vi "PM103 Peak Search Sample.vi"() -> ()   [LabVIEW 2019]
panel:
  out "Current [A]":string caption="Buffer"
  in  "Autoset":bool
  out "Active":bool
  in  "stop":bool
  # "Thorlabs Power Meter Series\n    PM103 peak search example"
  # "This example will connect the first found power meter."
  # "Connected"
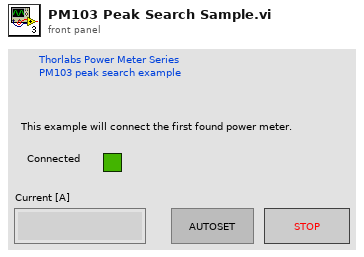
[diagram p1: front panel]
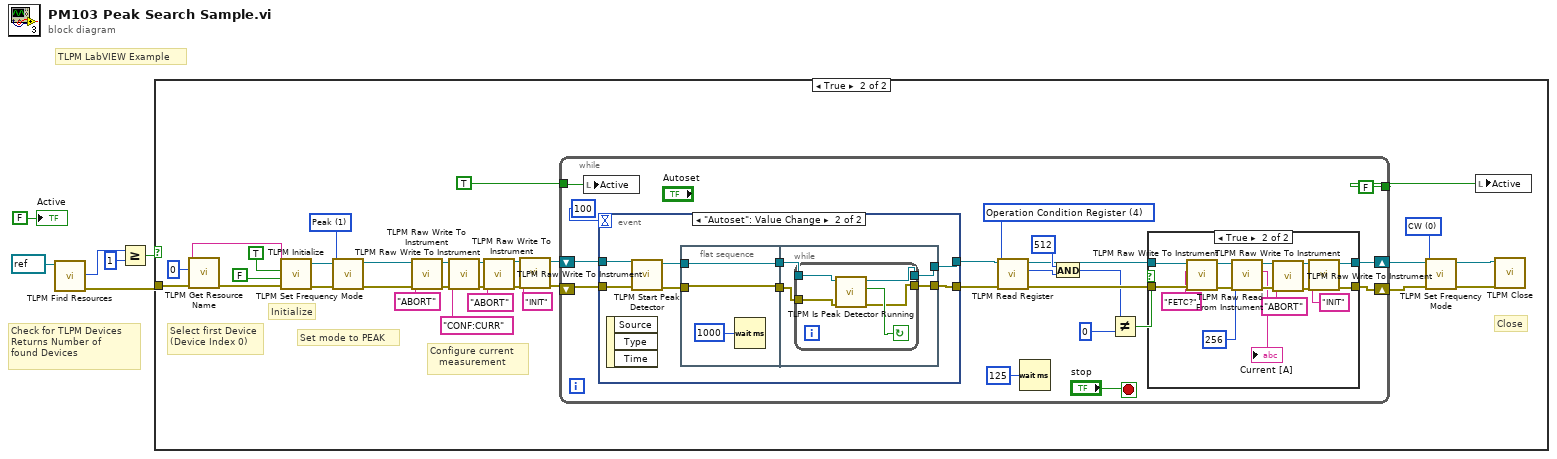
[diagram p0: block diagram]
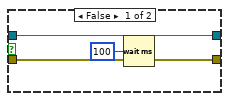
[diagram p3: hidden frame]
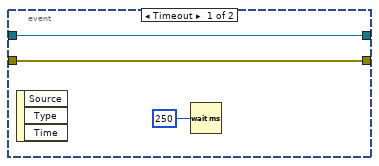
[diagram p4: hidden frame]
diagram:
  # "TLPM LabVIEW Example"
  # "Check for TLPM Devices\nReturns Number of\nfound Devices"
  n1 = call <instrlib>:"TLPM Find Resources.vi"("instrument handle"=refnum<visa-resource-name> refnum) -> ("error out"=w5:errorcluster, "Resource Count"=w3:u32)  [unwired: 8 in, 1 out]
  n2 = Greater Or Equal?(x=w3, y=u32 1) -> (x >= y?=w4:bool)
  n3 = case shown="True" w4 {
    tunnel: w5 -> [_ w34]
    frame False {
    }
    frame True {
      w7 = u16 1 items=["CW", "Peak"] ("Frequency Mode (Peak)")
      w24 = u16 0 items=["CW", "Peak"] ("Frequency Mode (Peak)")
      # "Configure current \n   measurement"
      # "Set mode to PEAK"
      # "Close"
      # "Initialize"
      # "Select first Device\n(Device Index 0)"
      n4 = call <instrlib>:"TLPM Get Resource Name.vi"("error in (no error)"=w34, "Index (0)"=u32 0 ("Device Index")) -> ("error out"=w36:errorcluster, "Resource Name"=w35:string)  [unwired: 7 in, 1 out]
      n5 = call <instrlib>:"TLPM Initialize.vi"("error in (no error)"=w36, "Reset Device (Reset Device)"=FALSE ("ID Query (Do Query)"), "ID Query (Do Query)"=TRUE, "resource name"=w35) -> ("error out"=w22:errorcluster, "instrument handle out"=w23:refnum<visa-resource-name>)  [unwired: 6 in]
      n6 = call <instrlib>:"TLPM Set Frequency Mode.vi"("error in (no error)"=w22, "Frequency Mode (Peak)"=w7, "instrument handle"=w23) -> ("error out"=w20:errorcluster, "instrument handle out"=w21:refnum<visa-resource-name>)  [unwired: 7 in]
      n7 = call <instrlib>:"TLPM Raw Write To Instrument.vi"("error in (no error)"=w20, "Command (\"*RST\")"="ABORT" ("Command (\"*RST\")"), "instrument handle"=w21) -> ("error out"=w19:errorcluster, "instrument handle out"=w13:refnum<visa-resource-name>)  [unwired: 7 in]
      n8 = call <instrlib>:"TLPM Raw Write To Instrument.vi"("error in (no error)"=w19, "Command (\"*RST\")"="CONF:CURR" ("Command (\"*RST\")"), "instrument handle"=w13) -> ("error out"=w18:errorcluster, "instrument handle out"=w12:refnum<visa-resource-name>)  [unwired: 7 in]
      n9 = call <instrlib>:"TLPM Raw Write To Instrument.vi"("error in (no error)"=w18, "Command (\"*RST\")"="ABORT" ("Command (\"*RST\")"), "instrument handle"=w12) -> ("error out"=w17:errorcluster, "instrument handle out"=w14:refnum<visa-resource-name>)  [unwired: 7 in]
      n10 = call <instrlib>:"TLPM Raw Write To Instrument.vi"("error in (no error)"=w17, "Command (\"*RST\")"="INIT" ("Command (\"*RST\")"), "instrument handle"=w14) -> ("error out"=w16:errorcluster, "instrument handle out"=w15:refnum<visa-resource-name>)  [unwired: 7 in]
      n11 = while {
        shift-right: [w42] -> w28
        shift-left: w15 -> [w50]
        shift-right: [w41] -> w27
        shift-left: w16 -> [w49]
        tunnel: [FALSE ("Active")] -> w32
        tunnel: TRUE ("Active") -> [w52]
        stop <- "stop" stop-if-true
        w48 = i16 4 items=["Status Byte Register"=0, "Service Request Enable"=1, "Standard Event Status Register"=2, "Standard Event Enable"=3, "Measurement Condition Register"=14, "Measurement Event Register"=15, "Measurement Event Enable Register"=16, "Measurement Positive Transition Filter"=17, "Measurement Negative Transition Filter"=18, "Operation Condition Register"=4, "Operation Event Register"=5, "Operation Event Enable Register"=6, "Operation Positive Transition Filter"=7, "Operation Negative Transition Filter"=8, "Questionable Condition Register"=9, "Questionable Event Register"=10, "Questionable Event Enable Register"=11, "Questionable Positive Transition Filter"=12, "Questionable Negative Transition Filter"=13, "Auxiliary Condition Register"=19, "Auxiliary Event Register"=20, "Auxiliary Event Enable Register"=21, "Auxiliary Positive Transition Filter"=22, "Auxiliary Negative Transition Filter"=23] ("Register ID (Status Byte Register)")
        n12 = local write "Active"(w52) -> ()
        n13 = event shown="[1] \"Autoset\": Value Change" {
          selector: _ -> [_ _]
          dyn-events: _ -> [_ _]
          timeout: 100 -> [_ _]
          tunnel: w50 -> [w75 w84]
          tunnel: w49 -> [w76 w83]
          tunnel: [w76 w78] -> w37
          tunnel: [w75 w77] -> w38
          event Timeout {
            n14 = event-data() -> ()  [unwired: 1 in, 3 out]
            n15 = Wait (ms)(milliseconds to wait=u32 250) -> ()  [unwired: 1 out]
          }
          event "Autoset": Value Change {
            n16 = event-data() -> ()  [unwired: 1 in, 3 out]
            n17 = call <instrlib>:"TLPM Start Peak Detector.vi"("error in (no error)"=w83, "instrument handle"=w84) -> ("error out"=w81:errorcluster, "instrument handle out"=w82:refnum<visa-resource-name>)  [unwired: 8 in]
            n18 = flat-sequence {
              tunnel: w82 -> [w86]
              tunnel: w81 -> [w85]
              tunnel: [w86] -> w80
              tunnel: [w85] -> w79
              tunnel: w80 -> [w91]
              tunnel: w79 -> [w90]
              tunnel: [w89] -> w78
              tunnel: [w88] -> w77
              frame #0 {
                n19 = Wait (ms)(milliseconds to wait=u32 1000) -> ()  [unwired: 1 out]
              }
              frame #1 {
                n20 = while {
                  tunnel: w91 -> [w93]
                  tunnel: w90 -> [w95]
                  tunnel: [w94] -> w89
                  tunnel: [w92] -> w88
                  stop <- w96 continue-if-true
                  n21 = call <instrlib>:"TLPM Is Peak Detector Running.vi"("error in (no error)"=w95, "instrument handle"=w93) -> ("error out"=w94:errorcluster, "Is Running"=w96:bool, "instrument handle out"=w92:refnum<visa-resource-name>)  [unwired: 7 in]
                }
              }
            }
          }
        }
        n22 = call <instrlib>:"TLPM Read Register.vi"("error in (no error)"=w37, "Register ID (Status Byte Register)"=w48, "instrument handle"=w38) -> ("error out"=w43:errorcluster, "Value"=w39:i16, "instrument handle out"=w44:refnum<visa-resource-name>)  [unwired: 6 in]
        n23 = Wait (ms)(milliseconds to wait=u32 125) -> ()  [unwired: 1 out]
        n24 = And(x=i16 512, y=w39) -> (x .and. y?=w40:i16)
        n25 = Not Equal?(x=w40, y=i16 0) -> (x != y?=w46:bool)
        n26 = case shown="True" w46 {
          tunnel: w44 -> [w57 w62]
          tunnel: w43 -> [w56 w73]
          tunnel: [w56 w65] -> w41
          tunnel: [w57 w64] -> w42
          frame False {
            n27 = Wait (ms)(milliseconds to wait=u32 100) -> ()  [unwired: 1 out]
          }
          frame True {
            n28 = call <instrlib>:"TLPM Raw Write To Instrument.vi"("error in (no error)"=w73, "Command (\"*RST\")"="FETC?" ("Command (\"*RST\")"), "instrument handle"=w62) -> ("error out"=w72:errorcluster, "instrument handle out"=w71:refnum<visa-resource-name>)  [unwired: 7 in]
            n29 = call <instrlib>:"TLPM Raw Read From Instrument.vi"("error in (no error)"=w72, "Size"=u32 256, "instrument handle"=w71) -> ("error out"=w66:errorcluster, "Buffer"=→"Current [A]":string, "instrument handle out"=w63:refnum<visa-resource-name>)  [unwired: 5 in, 1 out]
            n30 = call <instrlib>:"TLPM Raw Write To Instrument.vi"("error in (no error)"=w66, "Command (\"*RST\")"="ABORT" ("Command (\"*RST\")"), "instrument handle"=w63) -> ("error out"=w70:errorcluster, "instrument handle out"=w69:refnum<visa-resource-name>)  [unwired: 7 in]
            n31 = call <instrlib>:"TLPM Raw Write To Instrument.vi"("error in (no error)"=w70, "Command (\"*RST\")"="INIT" ("Command (\"*RST\")"), "instrument handle"=w69) -> ("error out"=w65:errorcluster, "instrument handle out"=w64:refnum<visa-resource-name>)  [unwired: 7 in]
          }
        }
      }
      n32 = call <instrlib>:"TLPM Set Frequency Mode.vi"("error in (no error)"=w27, "Frequency Mode (Peak)"=w24, "instrument handle"=w28) -> ("error out"=w26:errorcluster, "instrument handle out"=w25:refnum<visa-resource-name>)  [unwired: 7 in]
      n33 = local write "Active"(w32) -> ()
      n34 = call <instrlib>:"TLPM Close.vi"("error in (no error)"=w26, "instrument handle"=w25) -> ()  [unwired: 9 in, 1 out]
    }
  }
  "Active" <- FALSE ("Active")
